vi "section_parameters_cluster_to_writeable_section_parameters_cluster.vi"(8 "Error In":errorcluster, 11 "Section Parameters":T2) -> (0 "Error Out":errorcluster, 3 "Writeable Parameters":T1)   [LabVIEW 2019]
doc: "We can't write parameter clusters with paths and enums to file, so this converts that cluster to a writeable cluster."
uses:
  section_parameters_cluster_typedef.ctl
  sections_method_enum_typedef.ctl
  sections_edge_mode_enum_typedef.ctl
  sections_roi_size_enum_typedef.ctl
  xi_angles_enum_typedef.ctl
  writeable_section_parameters_cluster_typedef.ctl
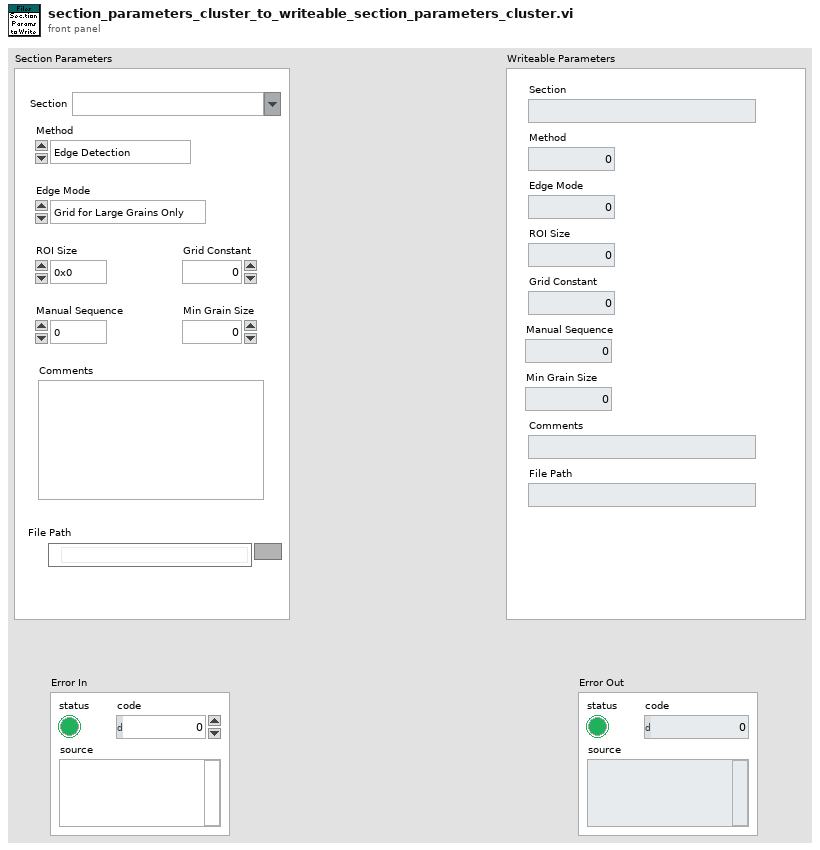
[diagram p1: front panel]
types:
  T1 = typedef "writeable_section_parameters_cluster_typedef.ctl" = cluster{"Section":string, "Method":i32, "Edge Mode":i32, "Grid Constant":i32, "Manual Sequence":i32, "ROI Size":i32, "Min Grain Size":dbl, "Comments":string, "File Path":string}
  T2 = typedef "section_parameters_cluster_typedef.ctl" = cluster{"Section":string, "Method":T3, "Edge Mode":T4, "ROI Size":T5, "Manual Sequence":T6, "Grid Constant":i32, "Min Grain Size":dbl, "Comments":string, "File Path":path}
  T3 = typedef "sections_method_enum_typedef.ctl" = enum16{"Edge Detection", "Grid Only", "Manual Selection", "Existing Edges"}
  T4 = typedef "sections_edge_mode_enum_typedef.ctl" = enum16{"Grid for Large Grains Only", "Grid", "No Grid"}
  T5 = typedef "sections_roi_size_enum_typedef.ctl" = enum16{"0x0", "1x1", "2x2", "3x3", "4x4", "5x5", "6x6"}
  T6 = typedef "xi_angles_enum_typedef.ctl" = enum16{"0", "45"}
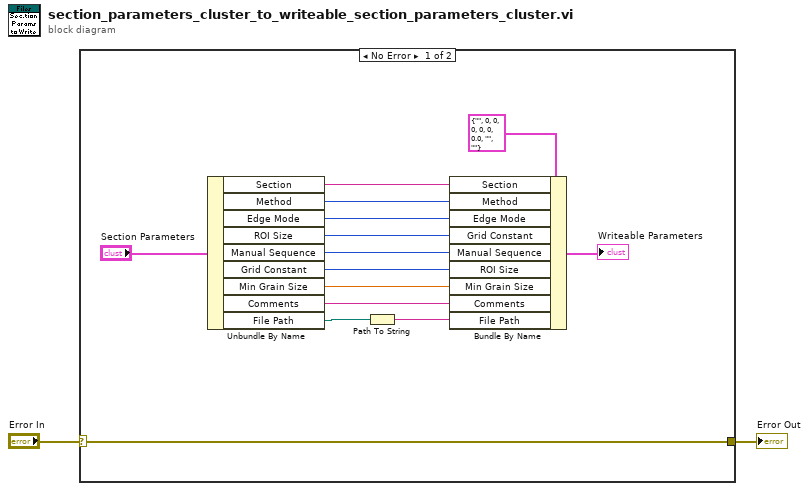
[diagram p0: block diagram]
diagram:
  n1 = case shown="No Error" "Error In" {
    selector: "Error In" -> [w16 w17]
    tunnel: [w16 w17] -> w1
    frame No Error {
      n2 = Unbundle By Name("Section Parameters") -> ("Section"=w13:string, "Method"=w12:T3, "Edge Mode"=w11:T4, "ROI Size"=w10:T5, "Manual Sequence"=w9:T6, "Grid Constant"=w8:i32, "Min Grain Size"=w7:dbl, "Comments"=w6:string, "File Path"=w5:path)
      n3 = Path To String(path=w5) -> (string=w4:string)
      n4 = Bundle By Name(cluster=T1 {"Section"="", "Method"=0, "Edge Mode"=0, "Grid Constant"=0, "Manual Sequence"=0, "ROI Size"=0, "Min Grain Size"=0.0, "Comments"="", "File Path"=""} ("Writeable Parameters"), "Section"=w13, "Method"=w12, "Edge Mode"=w11, "Grid Constant"=w10, "Manual Sequence"=w9, "ROI Size"=w8, "Min Grain Size"=w7, "Comments"=w6, "File Path"=w4) -> (→"Writeable Parameters":T1)
    }
    frame Error {
    }
  }
  "Error Out" <- w1
